vi "FM Voice Transmitter.vi"() -> ()   [LabVIEW 2013]
uses:
  <vilib>/sound2/lvsound2.llb/Sound File Info (path).vi
  <vilib>/sound2/lvsound2.llb/Sound File Read Open.vi
  <vilib>/Analysis/2dsp.llb/Rational Resample (single channel, DBL).vi
  <vilib>/sound2/lvsound2.llb/Sound File Read (DBL).vi
  <instrlib>/niUSRP/niUSRP Write Tx Data (CDB).vi
  <vilib>/Analysis/NI_AALPro.lvlib
panel:
  out "FM Waveform":dbl[](graph)
  in  "FM Deviation (Hz)":dbl(slide)=75000.0 scale=0.0..100000.0
  out "Waveform":waveform(dbl)(graph)
  in  "Path":path=path "E:/07/0416/let it go.wav"
  out "Constellation":cluster{dbl[], dbl[]}(graph)
  out "USRP Error Out":errorcluster
  out "Coerced Gain":dbl format="%#_6f"
  out "Coerced Carrier Freq.":dbl=2400010000.007024 format="%#_6p"
  out "Coerced IQ Rate":dbl=200000.0 format="%#_6p"
  in  "Stop":bool
  in  "Active Antenna":string="TX1"
  in  "Gain":dbl format="%#_6f"
  in  "Carrier Frequency":dbl=1200000000.0 format="%#_6p"
  in  "IQ Rate":dbl=200000.0 format="%#_6p"
  in  "Device Address":refnum<k15>="192.168.10.2"
  in  "Number of Samples":i32=44100
  # "FM Transmitter"
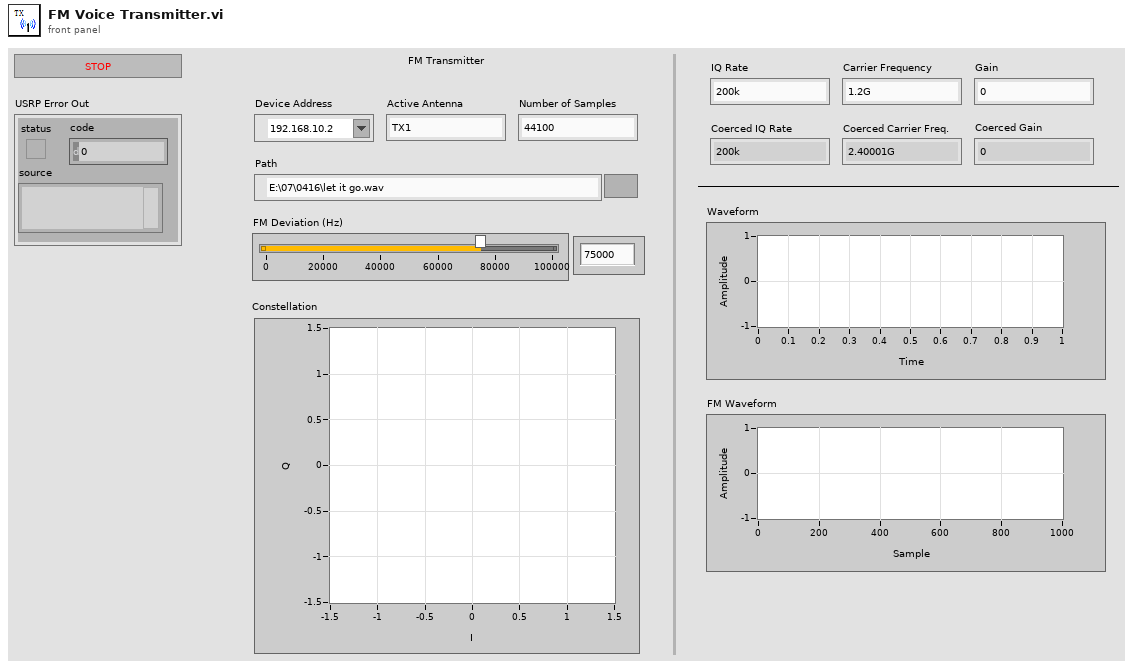
[diagram p1: front panel]
types:
  T1 = typedef "Sound Data Format.ctl" = cluster{"sample rate (S/s)":dbl, "number of channels":i32, "bits per sample":i32}
  T2 = typedef "Sound File Refnum.ctl" = refnum<file>
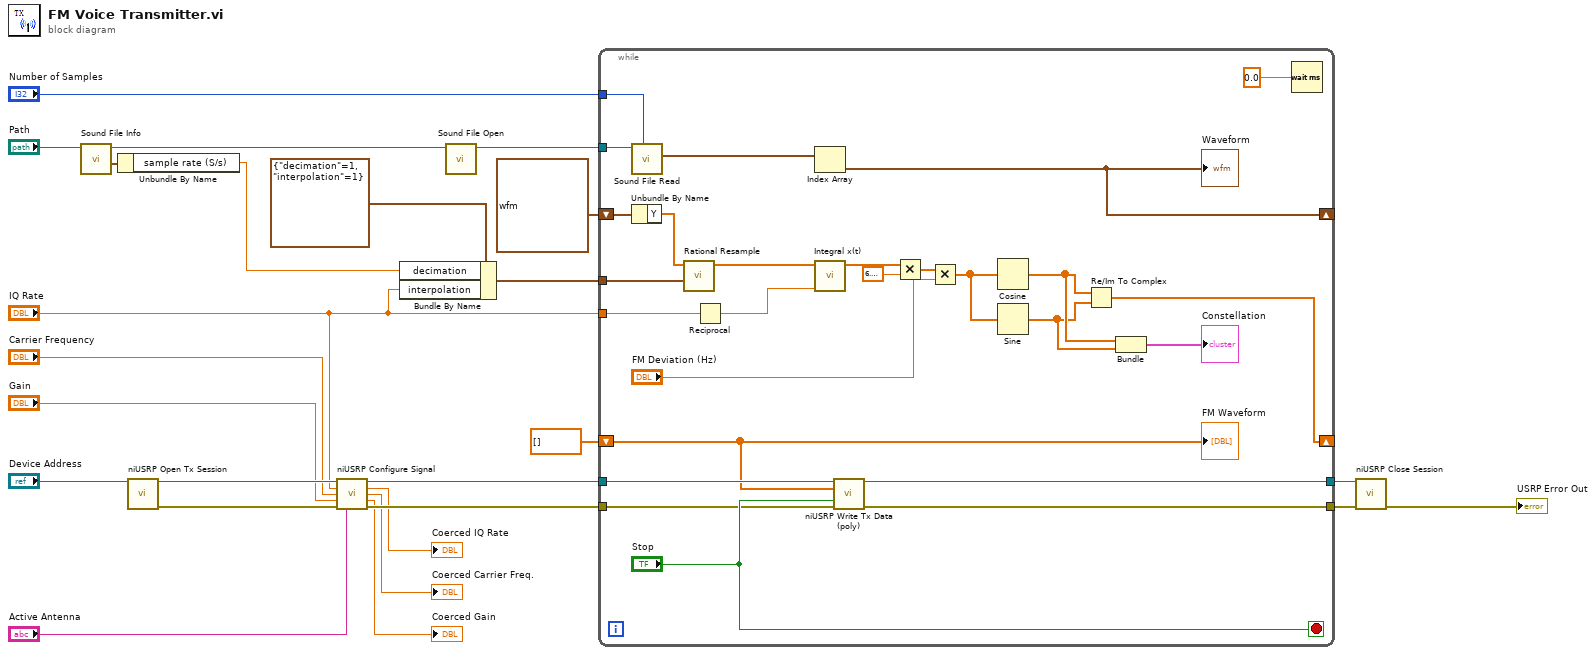
[diagram p0: block diagram]
diagram:
  n1 = call-poly <vilib>:"Sound File Info.vi"("path"="Path") -> ("sound format"=w14:T1, "path out"=w15:path)  [unwired: 7 in, 2 out]
  n2 = Unbundle By Name(w14) -> ("sample rate (S/s)"=w13:dbl)
  n3 = call <instrlib>:"niUSRP Open Tx Session.vi"("device names"="Device Address") -> ("session handle out"=w25:refnum<k15>, "error out"=w24:errorcluster)  [unwired: 13 in]
  n4 = call <instrlib>:"niUSRP Configure Signal.vi"("session handle"=w25, "IQ rate"="IQ Rate", "carrier frequency"="Carrier Frequency", "gain"="Gain", "error in (no error)"=w24, "active antenna"="Active Antenna") -> ("session handle out"=w22:refnum<k15>, "coerced IQ rate"=→"Coerced IQ Rate":dbl, "coerced carrier frequency"=→"Coerced Carrier Freq.":dbl, "coerced gain"=→"Coerced Gain":dbl, "error out"=w18:errorcluster)  [unwired: 5 in]
  n5 = Bundle By Name(cluster=cluster{"decimation":i32, "interpolation":i32} {"decimation"=1, "interpolation"=1}, "decimation"=w13, "interpolation"="IQ Rate") -> (w8:cluster{"decimation":i32, "interpolation":i32})
  n6 = call-poly <vilib>:"Sound File Open.vi"("path"=w15) -> ("sound file refnum"=w11:T2)  [unwired: 9 in, 1 out]
  n7 = while {
    tunnel: w22 -> [w51]
    shift-right: [w28] -> _
    shift-left: cdb[] [] -> [w26]
    tunnel: [w49] -> w20
    tunnel: [w48] -> w19
    tunnel: w18 -> [w47]
    tunnel: w11 -> [w46]
    tunnel: "Number of Samples" -> [w45]
    shift-right: [w43] -> _
    shift-left: waveform(dbl) {"t0"=timestamp(0 s since 1904-01-01), "dt"=1.0, "Y"=[]} ("Waveform") -> [w42]
    tunnel: w8 -> [w39]
    tunnel: "IQ Rate" -> [w38]
    stop <- "Stop" stop-if-true
    n8 = call-poly <vilib>:"Sound File Read.vi"("number of samples/ch (-1: all)"=w45, "sound file refnum"=w46) -> ("data"=w44:waveform(dbl)[])  [unwired: 5 in, 4 out]
    n9 = Unbundle By Name(w42) -> ("Y"=w41:dbl[])
    n10 = call-poly <vilib>:"Rational Resample.vi"("resample factor"=w39, "X"=w41) -> ("Y"=w40:dbl[])  [unwired: 7 in, 2 out]
    n11 = Reciprocal(x=w38) -> (1/x=w37:dbl)
    n12 = Index Array "Index Array"(array=w44) -> (element=w43:waveform(dbl))  [unwired: 1 in]
    "Waveform" <- w43
    n13 = call <vilib>:"Integral x(t).vi"("dt"=w37, "X"=w40) -> ("Integral X"=w36:dbl[])  [unwired: 8 in, 1 out]
    n14 = call-poly <instrlib>:"niUSRP Write Tx Data (poly).vi"("session handle"=w51, "data"=w26, "end of data?"="Stop", "error in (no error)"=w47) -> ("session handle out"=w49:refnum<k15>, "error out"=w48:errorcluster)  [unwired: 10 in]
    n15 = Multiply(x=w36, y=6.283185307179586) -> (x*y=w34:dbl[])
    n16 = Multiply(x=w34, y="FM Deviation (Hz)") -> (x*y=w32:dbl[])
    n17 = Cosine(x=w32) -> (cos(x)=w30:dbl[])
    n18 = Sine(x=w32) -> (sin(x)=w29:dbl[])
    n19 = Re/Im To Complex(1:w29, 2:w30) -> (0:w28:cdb[])
    n20 = Bundle(w30, w29) -> (→"Constellation":cluster{dbl[], dbl[]})  [unwired: 1 in]
    n21 = Wait (ms)(milliseconds to wait=0.0) -> ()  [unwired: 1 out]
    "FM Waveform" <- w26
  }
  n22 = call <instrlib>:"niUSRP Close Session.vi"("session handle"=w20, "error in (no error)"=w19) -> ("error out"=→"USRP Error Out":errorcluster)  [unwired: 13 in]
